vi "Write configuration.vi"(8 "error in (no error)":errorcluster, 11 "Murmex in":refnum<class "ExampleClassB.lvclass">) -> (0 "error out":errorcluster, 3 "Murmex out":refnum<class "ExampleClassB.lvclass">)   [LabVIEW 2012, in "ExampleClassB.lvclass"]
doc: "Writes the configuration cluster into the configuration file. Configuration file is XML-based. It's name is <component ID>.xml"
uses:
  ExampleClassB.lvclass
  <vilib>/Distrio/Murmex/Murmex/Murmex.lvclass
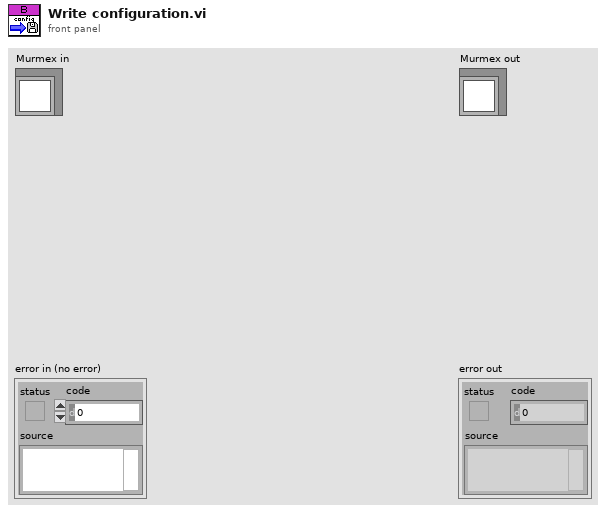
[diagram p1: front panel]
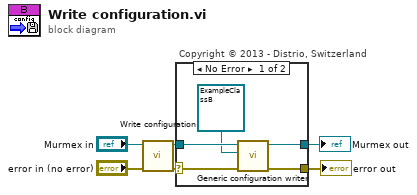
[diagram p0: block diagram]
diagram:
  n1 = call-parent "Write configuration.vi"("error in (no error)"="error in (no error)", "Murmex in"="Murmex in") -> ("error out"=w1:errorcluster, "Murmex out"=w3:refnum<class "ExampleClassB.lvclass">)  [unwired: 8 in]
  n2 = case "Copyright © 2013 - Distrio, Switzerland" shown="No Error" w1 {
    selector: w1 -> [w11 w13]
    tunnel: [w10 w13] -> w5
    tunnel: [w8 w12] -> w6
    tunnel: w3 -> [w9 w12]
    frame No Error {
      n3 = call <vilib>:"Generic configuration writer.vi"("error in (no error)"=w11, "inheritance level"=refnum<class "ExampleClassB.lvclass"> refnum ("ExampleClassB"), "Murmex in"=w9) -> ("error out"=w10:errorcluster, "Murmex out"=w8:refnum<class "ExampleClassB.lvclass">)  [unwired: 7 in]
    }
    frame Error {
    }
  }
  "error out" <- w5
  "Murmex out" <- w6
